vi "proptest_runtime class.vi"() -> ()   [LabVIEW 2013, in "NISE_CEF_Tests.lvlib"]
uses:
  Trunk/CEF_TreeControl/serializable configuration/NISE_CEF_serializable configuration.lvclass
  NISE_CEF_Tests.lvlib
panel:
  out "error 538305":errorcluster
  out "class name empty=ok":bool
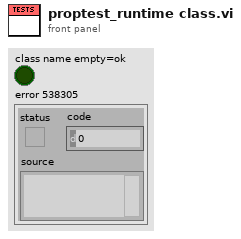
[diagram p1: front panel]
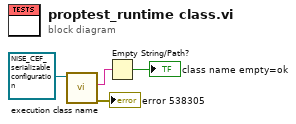
[diagram p0: block diagram]
diagram:
  n1 = call-dynamic "execution class name.vi"("configuration in"=refnum<class "NISE_CEF_serializable configuration.lvclass"> refnum ("configuration")) -> ("error out"=→"error 538305":errorcluster, "execution class"=w1:string)  [unwired: 8 in, 1 out]
  n2 = Empty String/Path?(string/path=w1) -> (empty?=→"class name empty=ok":bool)
